vi "Dashboard Main.vi"() -> ()   [LabVIEW 2017]
uses:
  <vilib>/Utility/miscctls.llb/LVRowAndColumnTypeDef.ctl
  <vilib>/event_ctls.llb/eventvkey.ctl
  <vilib>/Rock Robotics/Network Tables/NT Read Numeric Array.vi
  <vilib>/Rock Robotics/WPI/Dashboard/WPI_DashboardLogging Global.vi
panel:
  in  "Camera Settings Right":T1={"Frame Rate"=30, "Compression"=30, "Size"=1, "DB Camera Config"=FALSE} {"Frame Rate" scale=1.0..30.0; "Compression" scale=100.0..-1.0; "Size" items=["640x480", "320x240", "160x120"]}
  in  "Camera Name Right":string(combo)="No Camera Selection"
  out "Camera Info":cluster{"Mbps LED":bool, "Mbps":dbl, "fps":dbl} {"fps" format="%#.1g"; "Mbps" format="%#.1g"}
  in  "Camera Settings":T1={"Frame Rate"=30, "Compression"=30, "Size"=1, "DB Camera Config"=FALSE} {"Frame Rate" scale=1.0..30.0; "Compression" scale=100.0..-1.0; "Size" items=["640x480", "320x240", "160x120"]}
  in  "TCP":refnum<k5>
  in  "Rec Mode":enum32{"Stop", "Record", "Playback"}(radio)
  out "Robot IP":string
  out "Image Message":string="Timeout in Camera Communications"
  in  "Dashboard Tab":T2(tab)
  in  "Select Auto":string(combo)="Select Autonomous ..."
  out "NT Connection":bool
  out "MotorChart R":cluster{"Numeric":dbl, "Numeric":dbl}(graph)
  out "MotorChart L":cluster{"Numeric":dbl, "Numeric":dbl}(graph)
  out "MotorSliders R":cluster{"MotorSlide1":dbl, "MotorSlide2":dbl} {"MotorSlide2" scale=-1.0..1.0 scale format="%#_2e"; "MotorSlide1" scale=-1.0..1.0 scale format="%#_2e"}
  out "MotorSliders L":cluster{"MotorSlide1":dbl, "MotorSlide2":dbl} {"MotorSlide2" scale=-1.0..1.0 scale format="%#_2e"; "MotorSlide1" scale=-1.0..1.0 scale format="%#_2e"}
  out "Gyro":dbl(knob) scale=0.0..360.0
  out "JS1 Z":dbl(slide) scale=-1.0..1.0 scale format="%#_2e"
  out "JS1 Graph":cluster{"X":dbl, "Y":dbl}[](graph)
  out "JS1 Buttons":T3
  out "JS2 Z":dbl(slide) scale=-1.0..1.0 scale format="%#_2e"
  out "JS2 Graph":cluster{"X":dbl, "Y":dbl}[](graph)
  out "JS2 Buttons":T3
  out "Mode":T4(ring)=enum."Auto Disabled"
  out "Game Specific Data":string
  out "Camera Image Right":T5(plugin-control)
  in  "DB/String 9":string
  in  "DB/String 8":string
  in  "DB/String 7":string
  in  "DB/String 6":string
  in  "DB/String 5":string
  in  "DB/String 4":string
  in  "DB/String 3":string
  in  "DB/String 2":string
  in  "DB/String 1":string
  in  "DB/String 0":string
  in  "DB/Slider 0":dbl(slide) scale=0.0..5.0
  in  "DB/Slider 1":dbl(slide) scale=0.0..5.0
  in  "DB/Slider 2":dbl(slide) scale=0.0..5.0
  in  "DB/Slider 3":dbl(slide) scale=0.0..5.0
  out "DB/LED 3":bool
  out "DB/LED 2":bool
  out "DB/LED 1":bool
  out "DB/LED 0":bool
  in  "DB/Button 3":bool
  in  "DB/Button 2":bool
  in  "DB/Button 1":bool
  in  "DB/Button 0":bool caption="New Name"
  in  "Test Tune":bool
  out "Array":bool[][](array[boolean])
  in  "Test Slider":dbl(slide) scale=0.0..100.0 scale format="%#_3g"
  in  "On/Off":bool caption="Solenoid"
  in  "Test Name":u16(ring) items=["Select the test to run..."]
  in  "Test Tree":string(tree)
  in  "Motor":cluster{"Value":dbl, "Enable":bool} {"Value" scale=-1.0..1.0 scale format="%#_3g"}
  out "Progress":T6 {"Test Progress" scale=0.0..100.0}
  in  "Rev/Fwd":cluster{"Forward":bool, "Reverse":bool}
  in  "Test Ring":u16(ring) items=["Monochrome", "Color"]
  out "Cmd Status":string
  in  "Execute Command":bool
  in  "Command Params":string[][](table)
  in  "Command Selection":i32(listbox)
  in  "CheckList":i32(listbox)
  out "Tree":string(tree)
  out "Camera Image":T5(plugin-control)
  out "Background":bool
  in  "Camera Name":string(combo)="No Camera Selection"
  # "HW"
  # "HW"
  # "Joysticks"
  # "Drive Motors"
  # "Front"
  # "Right"
  # "Left"
  # "Back"
  # "This tab is a great place for autonomous settings and robot-specific values.\nPlace controls and indicators inside this tab and match name to\nDashboard Variables on robot. You can also delete this comment."
  # "Opponent Switch\nScale\nOwn Switch"
  # "Left\nRight"
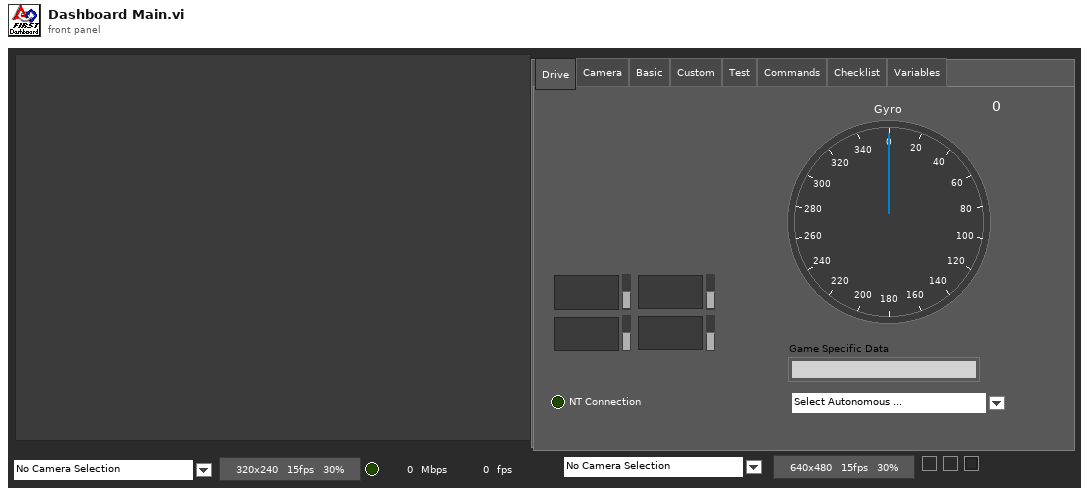
[diagram p1: front panel]
types:
  T1 = cluster{"Frame Rate":i32, "Compression":i32, "Size":u16, "DB Camera Config":bool}
  T2 = enum32{"Drive", "Camera", "Basic", "Custom", "Test", "Commands", "Checklist", "Variables"}
  T3 = cluster{bool, bool, bool, bool, bool, bool, bool, bool, bool, bool, bool, bool}
  T4 = enum8{"Tele-Op Disabled", "Tele-Op Enabled", "Auto Disabled", "Auto Enabled", "Test Disabled", "Test Enabled", "Disconnected", "No Code", "E-Stop"}
  T5 = typedef "IMAQ Image.ctl" = refnum<image>
  T6 = cluster{"Test Progress":u8, "Test Progress Text":string}
  T7 = cluster{"Save Path":path, "Interval (s)":dbl, "Keep":i32}
  T8 = typedef "Image Type" = u32
  T9 = cluster{"IDs":cluster{"RPC field ID":u16, "Unique ID":u16}, "String":string}
  T10 = cluster{"Error Strings":string, "Disable Counts":cluster{u16, u16}, "Rail Faults":cluster{u16, u16, u16}, "Robot IP":string, "DB Mode":u8, "Event Info":cluster{"Name":string, "Type":u8, "Number":u16, "Replay":u8}}
  T11 = cluster{"Storage":cluster{"Disk Free":u64, "RAM Block":u32, "RAM free":u32}, "CPU Utilization":cluster{"CPU % ISR":sgl, "CPU % Time Crit":sgl, "CPU % Timed Str":sgl, "CPU % High":sgl, "CPU % Above":sgl, "CPU % Normal":sgl, "CPU % Low":sgl}, "CAN":cluster{"% Bus Utilization":sgl, "Bus Off Cnt":u32, "TX_FIFO Full Cnt":u32, "Receive Error Cnt":u8, "Transmit Error Cnt":u8}, "HID":cluster{"HID Outputs":u32, "Rumble Low":u16, "Rumble High":u16}[]}
  T12 = cluster{"Status bits":cluster{"Test Mode":bool, "Autonomous":bool, "Enabled":bool, "Code Start":bool, "Brownout":bool, "Reserved 2":bool, "Reserved 3":bool, "E-Stop":bool}, "Code Trace":cluster{"Disabled":bool, "TeleOp":bool, "Auto":bool, "Test":bool}, "Controller Type":enum16{"unknown", "cRIO", "roboRio"}, "Code?":enum16{"unknown", "noCode", "code"}, "Battery V":dbl}
  T13 = cluster{"Control Bits":cluster{"TestMode":bool, "Autonomous":bool, "Enabled":bool, "FMS Present":bool, bool, bool, bool, "E-Stop":bool}, "Team Station ":u8, "Countdown":sgl, "Joystick Values":cluster{"Axes":dbl[], "Buttons":bool[], "POVs":i16[]}[]}
  T14 = cluster{"Axes":dbl[], "Buttons":bool[], "POVs":i16[]}[]
  T15 = cluster{"Axes":dbl[], "Buttons":bool[], "POVs":i16[]}
  T16 = cluster{"Buttons[0]":bool, "Buttons[1]":bool, "Buttons[2]":bool, "Buttons[3]":bool, "Buttons[4]":bool, "Buttons[5]":bool, "Buttons[6]":bool, "Buttons[7]":bool, "Buttons[8]":bool, "Buttons[9]":bool, "Buttons[10]":bool, "Buttons[11]":bool}
  T17 = cluster{"Camera Image":refnum<vi>, "Dashboard Tab":refnum<vi>, "Background":refnum<vi>, "Rec Mode":refnum<vi>, "Test Slider":refnum<vi>, "On/Off ":refnum<vi>, "Test Ring":refnum<vi>, "Rev/Fwd":refnum<vi>, "Test Name":refnum<vi>, "Motor":refnum<vi>, "Progress":refnum<vi>, "CheckList":refnum<vi>, "Tree":refnum<vi>, "Test Tree":refnum<vi>, "Command Params":refnum<vi>, "Command Selection":refnum<vi>, "Execute Command":refnum<vi>, "Cmd Status":refnum<vi>, "Camera Settings":refnum<vi>, "Camera Name":refnum<vi>, "Camera Info":refnum<vi>, "Camera Settings Right":refnum<vi>, "Camera Name Right":refnum<vi>, "Camera Image Right":refnum<vi>}
  T18 = cluster{"Camera Name":string, string, "Saved DB Images Info":cluster{"Save Path":path, "Interval (s)":dbl, "Keep":i32}}
  T19 = cluster{"Camera Name Right":string, string, "Saved DB Images Info":cluster{"Save Path":path, "Interval (s)":dbl, "Keep":i32}}
  T20 = cluster{"Operation":enum16{"Update", "Clear"}, "Color Box":u32}[]
  T21 = typedef "eventvkey.ctl" = enum16{"ASCII", "Enter", "Return", "Shift", "Ctrl", "Alt", "Cmd", "Opt", "Caps", "NumLock", "Clear", "Break", "Up", "Down", "Left", "Right", "Insert", "Delete", "Home", "End", "PageUp", "PageDown", "Escape", "Help", "Pause", "ScrollLock", "F1", "F2", "F3", "F4", "F5", "F6", "F7", "F8", "F9", "F10", "F11", "F12", "F13", "F14", "F15", "F16", "F17", "F18", "F19", "F20", "F21", "F22", "F23", "F24", "Play", "VolumeUp", "VolumeDown", "Mute", "Two Byte Char"}
  T22 = cluster{"Image Size":bool, "Image Type":bool, "Pixel Value":bool, "ROI Information":bool, "Zoom Factor":bool}
  T23 = cluster{"Operation":enum16{"Update", "Clear"}, "Color Box":u32}
  T24 = typedef "LVRowAndColumnTypeDef.ctl" = cluster{"Row":i32, "Column":i32}
  T25 = cluster{"Shift":bool, "Ctrl":bool, "Alt":bool, "Cmd":bool, "Opt":bool}
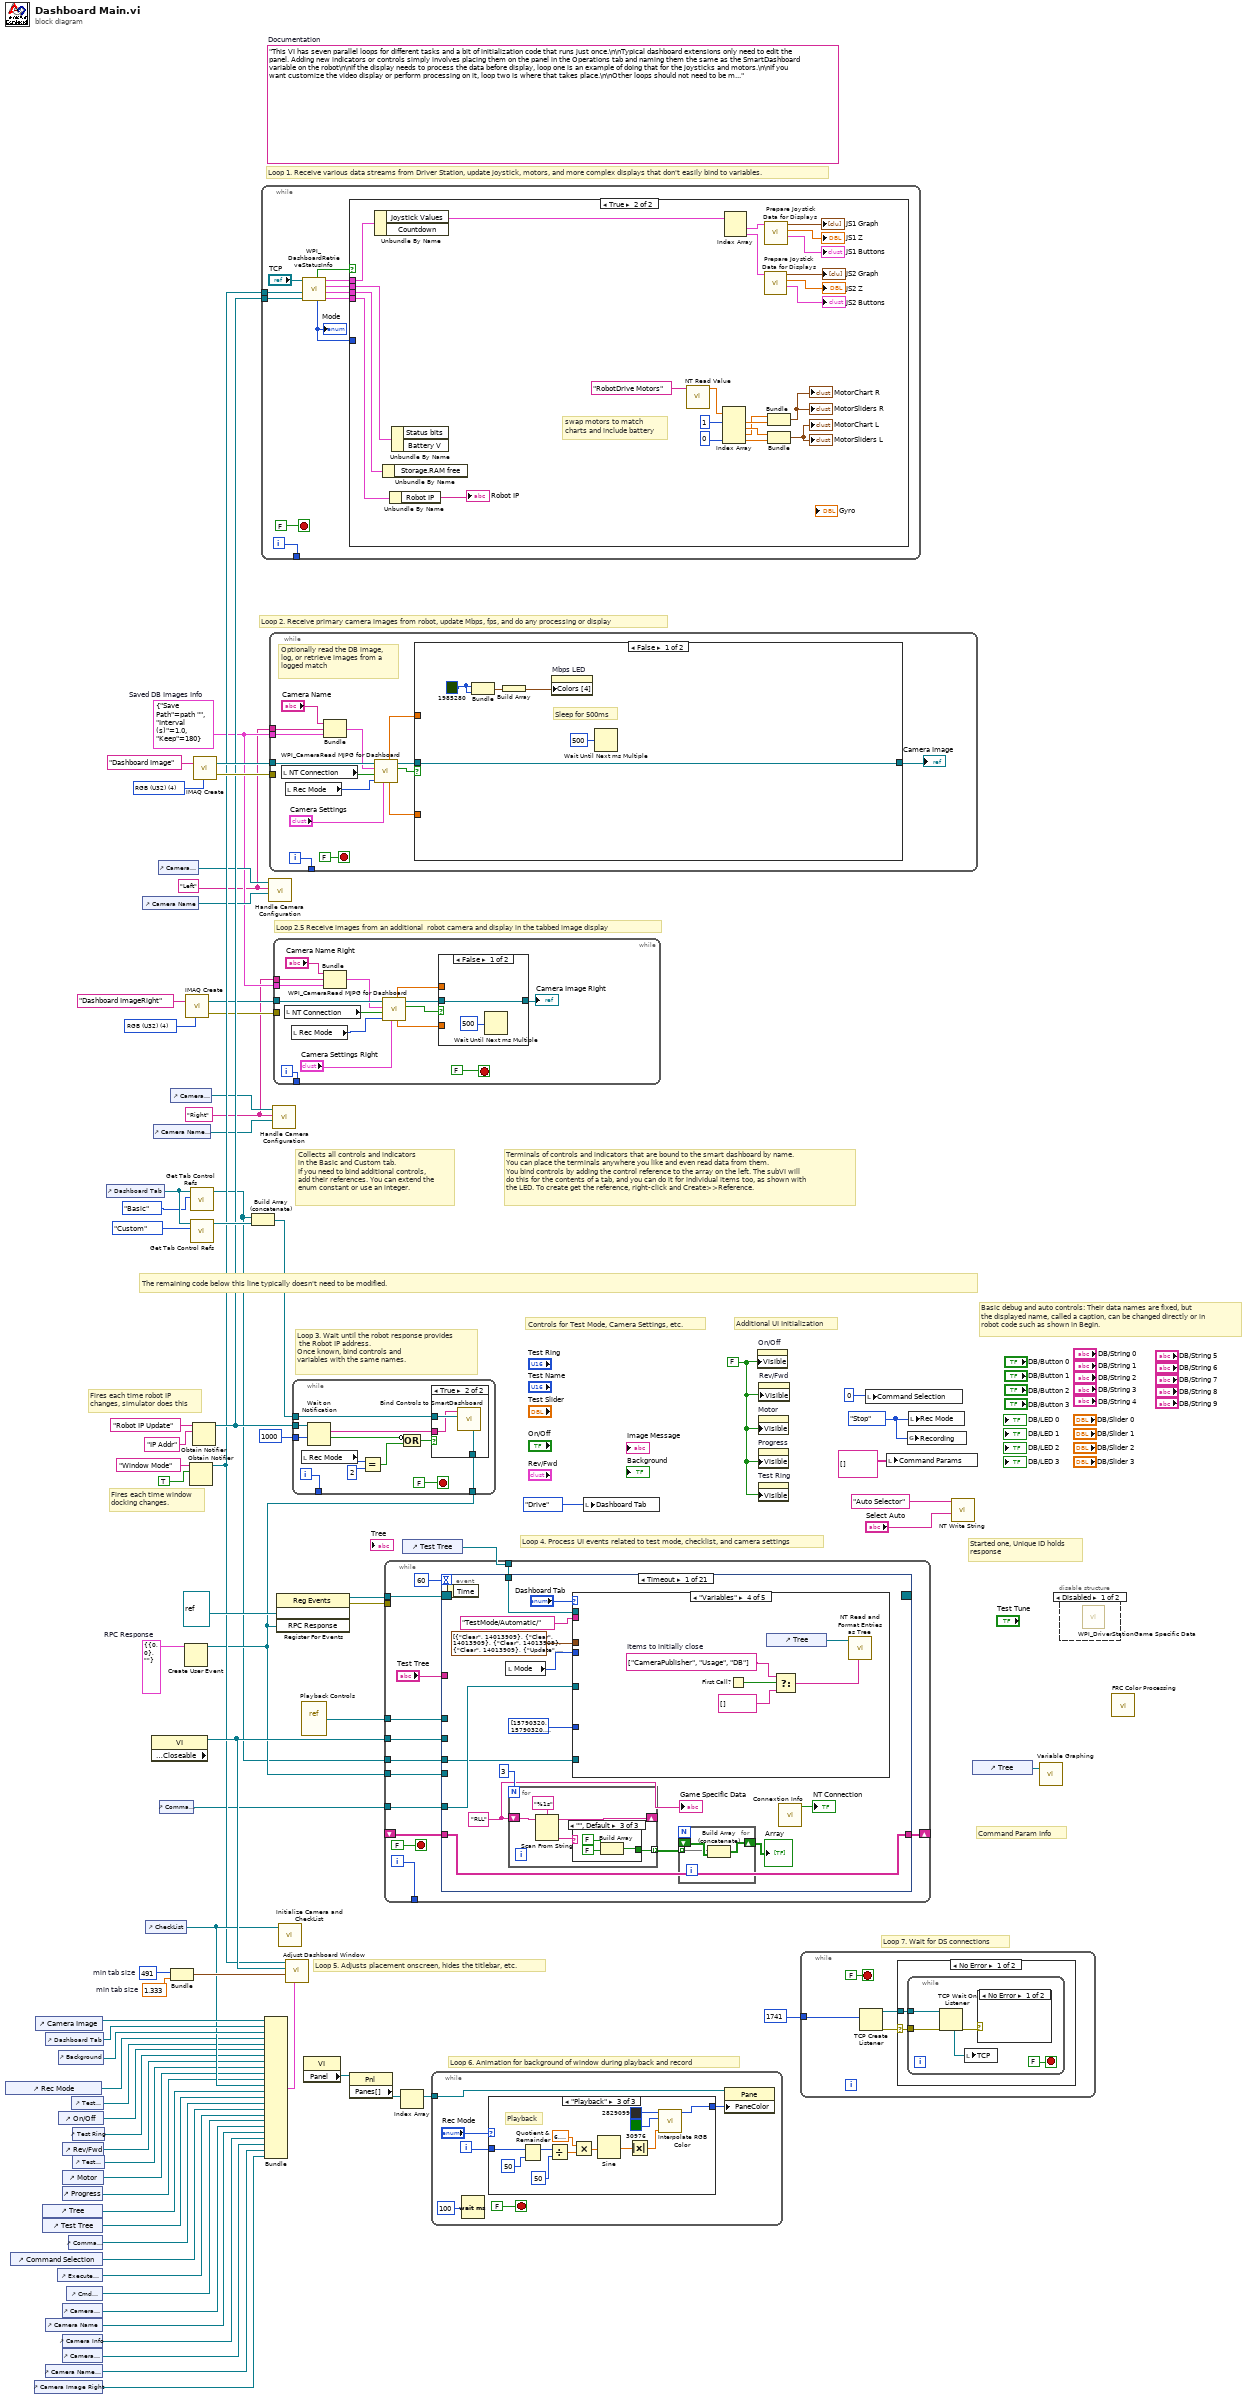
[diagram p0: block diagram]
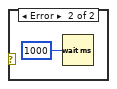
[diagram p4: hidden frame]
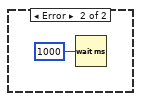
[diagram p5: hidden frame]
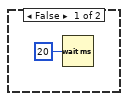
[diagram p6: hidden frame]
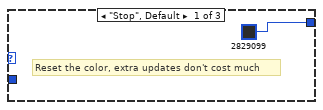
[diagram p7: hidden frame]
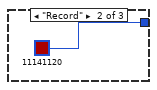
[diagram p8: hidden frame]
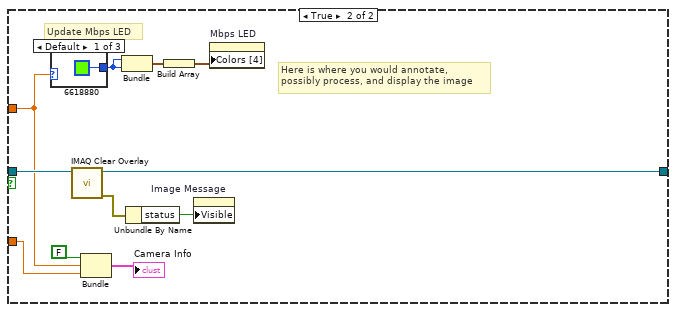
[diagram p10: hidden frame]
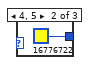
[diagram p11: hidden frame]
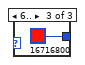
[diagram p12: hidden frame]
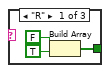
[diagram p13: hidden frame]
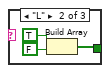
[diagram p14: hidden frame]
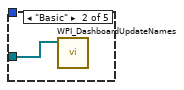
[diagram p16: hidden frame]
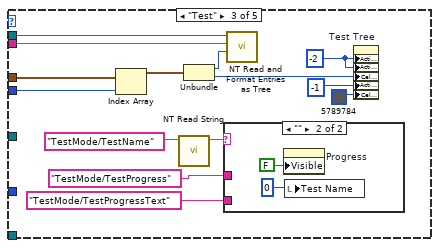
[diagram p17: hidden frame]
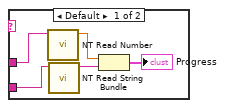
[diagram p18: hidden frame]
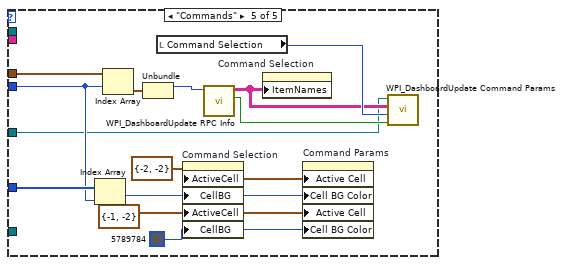
[diagram p19: hidden frame]
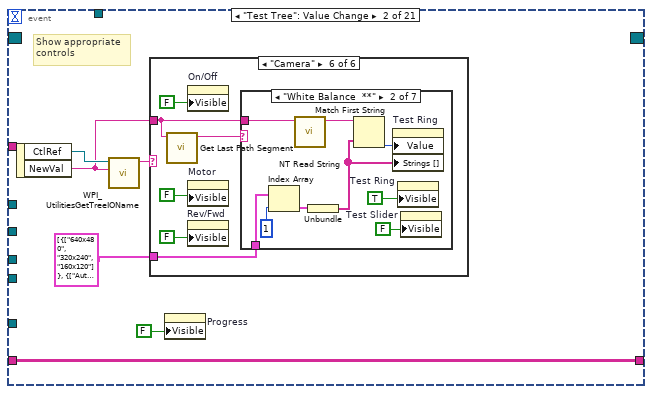
[diagram p20: hidden frame]
diagram:
  w4 = T7 {"Save Path"=path "", "Interval (s)"=1.0, "Keep"=180}  # Saved DB Images Info
  w3 = "Right"
  w2 = "Left"
  w14 = T8 4 items=["Grayscale (U8)", "Grayscale (I16)", "Grayscale (SGL)", "Complex (CSG)", "RGB (U32)", "HSL (U32)", "RGB (U64)"] ("Image Type")
  w30 = T9 {"IDs"={"RPC field ID"=0, "Unique ID"=0}, "String"=""}  # RPC Response
  w53 = 491  # min tab size
  w52 = 1.333  # min tab size
  w60 = enum32{"Stop", "Record", "Playback"}."Stop" ("Rec Mode")
  w37 = FALSE ("Visible")
  (unwired) "This VI has seven parallel loops for different tasks and a bit of initialization code that runs just once.\n\nTypical dashboard extensions only need to edit the panel. Adding new indicators or controls simply involves placing them on the panel in the Operations tab and naming them the same as the SmartDashboard variable on the robot\n\nIf the display needs to process the data before display, loop one is an example of doing that for the joysticks and motors.\n\nIf you want customize the video display or perform processing on it, loop two is where that takes place.\n\nOther loops should not need to be modified. They are pretty standard, and document the task they perform."  # Documentation
  w77 = T8 4 items=["Grayscale (U8)", "Grayscale (I16)", "Grayscale (SGL)", "Complex (CSG)", "RGB (U32)", "HSL (U32)", "RGB (U64)"] ("Image Type")
  # "Loop 2.5 Receive images from an additional  robot camera and display in the tabbed image display"
  # "Command Param Info"
  # "Started one, Unique ID holds\nresponse"
  # "Loop 7. Wait for DS connections"
  # "Basic debug and auto controls: Their data names are fixed, but\nthe displayed name, called a caption, can be changed directly or in\nrobot code such as shown in Begin."
  # "Controls for Test Mode, Camera Settings, etc."
  # "Additional UI Initialization"
  # "Loop 6. Animation for background of window during playback and record"
  # "Fires each time robot IP\nchanges, simulator does this"
  # "Fires each time window\ndocking changes."
  # "Collects all controls and indicators\nin the Basic and Custom tab.\nIf you need to bind additional controls,\nadd their references. You can extend the\nenum constant or use an integer."
  # "The remaining code below this line typically doesn't need to be modified."
  # "Loop 4. Process UI events related to test mode, checklist, and camera settings"
  # "Terminals of controls and indicators that are bound to the smart dashboard by name.\nYou can place the terminals anywhere you like and even read data from them.\nYou bind controls by adding the control reference to the array on the left. The subVI will\ndo this for the contents of a tab, and you can do it for individual items too, as shown with\nthe LED. To create get the reference, right-click and Create>>Reference."
  # "Loop 3. Wait until the robot response provides\n the Robot IP address.\nOnce known, bind controls and\nvariables with the same names."
  # "Loop 5. Adjusts placement onscreen, hides the titlebar, etc."
  # "Loop 1. Receive various data streams from Driver Station, update joystick, motors, and more complex displays that don't easily bind to variables."
  # "Loop 2. Receive primary camera images from robot, update Mbps, fps, and do any processing or display"
  n1 = control-ref of="Rec Mode"() -> (w43:refnum<vi>)
  n2 = control-ref of="Command Selection"() -> (w29:refnum<vi>)
  n3 = control-ref of="Camera Image Right"() -> (w7:refnum<vi>)
  n4 = control-ref of="Camera Image"() -> (w55:refnum<vi>)
  n5 = control-ref of="Tree"() -> (w47:refnum<vi>)
  n6 = control-ref of="Test Tree"() -> (w46:refnum<vi>)
  n7 = control-ref of="Dashboard Tab"() -> (w54:refnum<vi>)
  n8 = control-ref of="Camera Name"() -> (w20:refnum<vi>)
  n9 = control-ref of="Camera Name Right"() -> (w8:refnum<vi>)
  n10 = control-ref of="Execute Command"() -> (w31:refnum<vi>)
  n11 = control-ref of="Background"() -> (w50:refnum<vi>)
  n12 = control-ref of="On/Off"() -> (w41:refnum<vi>)
  n13 = control-ref of="Progress"() -> (w38:refnum<vi>)
  n14 = control-ref of="Camera Settings"() -> (w21:refnum<vi>)
  n15 = control-ref of="Camera Info"() -> (w19:refnum<vi>)
  n16 = control-ref of="Camera Settings Right"() -> (w9:refnum<vi>)
  n17 = control-ref of="Rev/Fwd"() -> (w39:refnum<vi>)
  n18 = control-ref of="Motor"() -> (w44:refnum<vi>)
  n19 = control-ref of="Cmd Status"() -> (w25:refnum<vi>)
  n20 = control-ref of="Command Params"() -> (w32:refnum<vi>)
  n21 = control-ref of="Test Slider"() -> (w42:refnum<vi>)
  n22 = control-ref of="Test Ring"() -> (w40:refnum<vi>)
  n23 = control-ref of="Test Name"() -> (w45:refnum<vi>)
  n24 = control-ref of="Dashboard Tab"() -> (w58:refnum<vi>)
  n25 = control-ref of="Camera Name"() -> (w22:refnum<vi>)
  n26 = control-ref of="CheckList"() -> (w48:refnum<vi>)
  n27 = property class="VI" props=["Front Panel.Closeable"]() -> (reference out=w59:refnum<vi>)  [unwired: 2 in, 2 out]
  n28 = control-ref of="Camera Name Right"() -> (w10:refnum<vi>)
  n29 = control-ref of="Camera Settings"() -> (w23:refnum<vi>)
  n30 = control-ref of="Command Params"() -> (w24:refnum<vi>)
  n31 = control-ref of="Camera Settings Right"() -> (w11:refnum<vi>)
  n32 = Bundle("min tab size"=w53, "min tab size"=w52) -> (w51:cluster{"min tab size":i32, "min tab size":dbl})  [unwired: 1 in]
  n33 = Create User Event(user event datatype=w30) -> (user event=w26:refnum<user-event>)  [unwired: 1 in, 1 out]
  n34 = call "IMAQ Create"("Image Name"="Dashboard ImageRight", "Image Type"=w14) -> ("New Image"=w13:T5, "error out"=w12:errorcluster)  [unwired: 2 in, 1 out]
  n35 = Obtain Notifier(name (unnamed)="Window Mode", notification data type=TRUE) -> (notifier out=w35:refnum<notifier>)  [unwired: 2 in, 2 out]
  n36 = call <vilib>:"Get Tab Control Refs.vi"("Page Index"=T2."Basic" ("Dashboard Tab"), "TabControl in"=w58) -> ("ControlsOnPage"=w18:refnum<vi>[])  [unwired: 9 in]
  n37 = call <vilib>:"Get Tab Control Refs.vi"("Page Index"=T2."Custom" ("Dashboard Tab"), "TabControl in"=w58) -> ("ControlsOnPage"=w57:refnum<vi>[])  [unwired: 9 in]
  n38 = Obtain Notifier(name (unnamed)="Robot IP Update", notification data type="IP Addr" ("name (unnamed)")) -> (notifier out=w36:refnum<notifier>)  [unwired: 2 in, 2 out]
  n39 = call "IMAQ Create"("Image Name"="Dashboard Image", "Image Type"=w77) -> ("New Image"=w75:T5, "error out"=w74:errorcluster)  [unwired: 2 in, 1 out]
  n40 = Build Array (concatenate)(w18, w57) -> (w56:refnum<vi>[])
  n41 = while {
    tunnel: [w87] -> _
    tunnel: w36 -> [w81]
    tunnel: w35 -> [w78]
    i -> [w87]
    stop <- FALSE stop-if-true
    n42 = call <vilib>:"WPI_DashboardRetrieveStatusInfo.vi"("Binding Refnum"=w81, "Window Mode Notifier"=w78, "TCP Cnx"="TCP") -> ("Power and Errors"=w82:T10, "Robot Metrics"=w85:T11, "Status Info"=w86:T12, "Control Info"=w83:T13, "Robot Mode"=w80:T4, "Process?"=w84:bool)  [unwired: 3 in]
    "Mode" <- w80
    n43 = case shown="True" w84 {
      tunnel: w86 -> [_ w113]
      tunnel: w85 -> [_ w112]
      tunnel: w83 -> [_ w111]
      tunnel: w82 -> [_ w110]
      tunnel: w80 -> [_ _]
      frame False {
        n44 = Wait (ms)(milliseconds to wait=u32 20) -> ()  [unwired: 1 out]
      }
      frame True {
        # "swap motors to match\ncharts and include battery"
        n45 = Unbundle By Name(w111) -> ("Joystick Values"=w101:T14)  [unwired: 1 out]
        n46 = Unbundle By Name(w112) -> ()  [unwired: 1 out]
        n47 = Unbundle By Name(w110) -> ("Robot IP"=→"Robot IP":string)
        n48 = Unbundle By Name(w113) -> ()  [unwired: 2 out]
        n49 = call-poly <vilib>:"NT Read Value.vi"("Name"="RobotDrive Motors") -> ("Numeric Array"=w91:dbl[])  [unwired: 9 in, 1 out]
        n50 = Index Array(array=w91, index #1=1, index #4=0) -> (element #1=w105:dbl, element #2=w106:dbl, element #3=w104:dbl, element #4=w109:dbl)  [unwired: 2 in]
        n51 = Index Array(array=w101) -> (element #1=w100:T15, element #2=w96:T15)  [unwired: 2 in]
        n52 = call "Prepare Joystick Data for Displays.vi"("Joystick Values"=w96) -> ("Buttons"=→"JS2 Buttons":T16, "Z Axis"=→"JS2 Z":dbl, "Cartesian Data"=→"JS2 Graph":cluster{"X axis":dbl, "X axis":dbl}[])  [unwired: 8 in]
        n53 = call "Prepare Joystick Data for Displays.vi"("Joystick Values"=w100) -> ("Buttons"=→"JS1 Buttons":T16, "Z Axis"=→"JS1 Z":dbl, "Cartesian Data"=→"JS1 Graph":cluster{"X axis":dbl, "X axis":dbl}[])  [unwired: 8 in]
        n54 = Bundle("Numeric"=w104, "Numeric"=w105) -> (→"MotorChart R" →"MotorSliders R":cluster{"Numeric":dbl, "Numeric":dbl})  [unwired: 1 in]
        n55 = Bundle("Numeric"=w106, "Numeric"=w109) -> (→"MotorChart L" →"MotorSliders L":cluster{"Numeric":dbl, "Numeric":dbl})  [unwired: 1 in]
      }
    }
  }
  n56 = Bundle("Camera Image"=w55, "Dashboard Tab"=w54, "Background"=w50, "Rec Mode"=w43, "Test Slider"=w42, "On/Off"=w41, "Test Ring"=w40, "Rev/Fwd"=w39, "Test Name"=w45, "Motor"=w44, "Progress"=w38, "CheckList"=w48, "Tree"=w47, "Test Tree"=w46, "Command Params"=w32, "Command Selection"=w29, "Execute Command"=w31, "Cmd Status"=w25, "Camera Settings"=w21, "Camera Name"=w20, "Camera Info"=w19, "Camera Settings Right"=w9, "Camera Name Right"=w8, "Camera Image Right"=w7) -> (w49:T17)  [unwired: 1 in]
  n57 = call "Handle Camera Configuration.vi"("CameraNameRef"=w22, "Display Name"=w2, "ClusterRef"=w23) -> ()  [unwired: 9 in]
  n58 = while {
    tunnel: w75 -> [w126]
    tunnel: w74 -> [_]
    tunnel: [w127] -> _
    tunnel: w4 -> [w117]
    tunnel: w2 -> [w114]
    i -> [w127]
    stop <- FALSE stop-if-true
    # "Optionally read the DB image,\nlog, or retrieve images from a\nlogged match"
    n59 = local read "NT Connection"() -> (w118:bool)
    n60 = local read "Rec Mode"() -> (w122:enum32{"Stop", "Record", "Playback"})
    n61 = Bundle("Camera Name"="Camera Name", w114, "Saved DB Images Info"=w117) -> (w116:T18)  [unwired: 1 in]
    n62 = call <vilib>:"WPI_CameraRead MJPG for Dashboard.vi"("Camera Settings"="Camera Settings", "Rec Mode"=w122, "NT Connection"=w118, "Capture Info"=w116, "Refnum in"=w126) -> ("Active"=w124:bool, "Refnum out"=w125:T5, "FPS"=w123:dbl, "Bandwidth (Mbps)"=w121:dbl)  [unwired: 3 in]
    n63 = case shown="False" w124 {
      tunnel: w125 -> [w129 w140]
      tunnel: w121 -> [_ w137]
      tunnel: w123 -> [_ w138]
      tunnel: [w129 w134] -> w119
      frame False {
        w131 = u32 1985280 ("Color Box")
        # "Sleep for 500ms"
        n64 = Bundle("Color Box"=w131, "Color Box"=w131) -> (w132:cluster{"Color Box":u32, "Color Box":u32})  [unwired: 1 out]
        n65 = Build Array(w132) -> (w130:cluster{"Color Box":u32, "Color Box":u32}[])
        n66 = property on="Mbps LED" class="Bool (strict)"("Colors [4]"=w130) -> ()  [unwired: 2 in, 2 out]
        n67 = Wait Until Next ms Multiple(millisecond multiple=u32 500) -> ()  [unwired: 1 out]
      }
      frame True {
        # "Here is where you would annotate,\npossibly process, and display the image"
        # "Update Mbps LED"
        n68 = case shown="Default" w137 {
          tunnel: [u32 6618880 ("Color Box") u32 16776722 ("Color Box") u32 16716800 ("Color Box")] -> w141
          frame Default {
          }
          frame 4, 5 {
          }
          frame 6.. {
          }
        }
        n69 = call "IMAQ Clear Overlay"("Image"=w140) -> ("error out"=w143:errorcluster, "Image Out"=w134:T5)  [unwired: 2 in, 7 out]
        n70 = Bundle(FALSE, "Bandwidth (Mbps)"=w137, "FPS"=w138) -> (→"Camera Info":cluster{bool, "Bandwidth (Mbps)":dbl, "FPS":dbl})  [unwired: 1 in]
        n71 = Bundle("Color Box"=w141, "Color Box"=w141) -> (w142:cluster{"Color Box":u32, "Color Box":u32})  [unwired: 1 out]
        n72 = Unbundle By Name(w143) -> ("status"=w144:bool)
        n73 = Build Array(w142) -> (w139:cluster{"Color Box":u32, "Color Box":u32}[])
        n74 = property on="Image Message" class="Str"("Visible"=w144) -> ()  [unwired: 2 in, 2 out]
        n75 = property on="Mbps LED" class="Bool (strict)"("Colors [4]"=w139) -> ()  [unwired: 2 in, 2 out]
      }
    }
    "Camera Image" <- w119
  }
  n76 = call "Handle Camera Configuration.vi"("CameraNameRef"=w10, "Display Name"=w3, "ClusterRef"=w11) -> ()  [unwired: 9 in]
  n77 = while {
    tunnel: w13 -> [w162]
    tunnel: w12 -> [_]
    tunnel: [w157] -> _
    tunnel: w4 -> [w151]
    tunnel: w3 -> [w148]
    i -> [w157]
    stop <- FALSE stop-if-true
    n78 = local read "NT Connection"() -> (w152:bool)
    n79 = local read "Rec Mode"() -> (w161:enum32{"Stop", "Record", "Playback"})
    n80 = Bundle("Camera Name Right"="Camera Name Right", w148, "Saved DB Images Info"=w151) -> (w150:T19)  [unwired: 1 in]
    n81 = call <vilib>:"WPI_CameraRead MJPG for Dashboard.vi"("Camera Settings"="Camera Settings Right", "Rec Mode"=w161, "NT Connection"=w152, "Capture Info"=w150, "Refnum in"=w162) -> ("Active"=w156:bool, "Refnum out"=w159:T5, "FPS"=w154:dbl, "Bandwidth (Mbps)"=w155:dbl)  [unwired: 3 in]
    n82 = case shown="False" w156 {
      tunnel: w159 -> [w163 w165]
      tunnel: w155 -> [_ _]
      tunnel: w154 -> [_ _]
      tunnel: [w163 w165] -> w153
      frame False {
        n83 = Wait Until Next ms Multiple(millisecond multiple=u32 500) -> ()  [unwired: 1 out]
      }
      frame True {
      }
    }
    "Camera Image Right" <- w153
  }
  n84 = register-events(refnum<vi> refnum, w26) -> (reference out=w64:refnum<event-registration>, error out=w63:errorcluster)  [unwired: 2 in]
  n85 = call "Initialize Camera and CheckList.vi"("ListBox in"=w48) -> ()  [unwired: 11 in]
  n86 = call "Adjust Dashboard Window.vi"("Sizing Refnums"=w49, "Size Constraints"=w51, "VI"=w59, "WIn Mode"=w35) -> ()  [unwired: 8 in]
  n87 = while {
    tunnel: w56 -> [w177]
    tunnel: w36 -> [w175]
    tunnel: [w173] -> _
    tunnel: u32 1000 ("milliseconds to wait") -> [w172]
    tunnel: w26 -> [w166]
    i -> [w173]
    stop <- FALSE stop-if-true
    n88 = local read "Rec Mode"() -> (w168:enum32{"Stop", "Record", "Playback"})
    n89 = Wait on Notification(notifier=w175, timeout in ms (-1)=w172) -> (notification=w174:string, timed out?=w170:bool)  [unwired: 2 in, 2 out]
    n90 = Equal?(x=w168, y=u16 2 ("Rec Mode")) -> (x = y?=w169:bool)
    n91 = Compound Arithmetic op=OR(invert w170, w169) -> (w171:bool)
    n92 = case shown="True" w171 {
      tunnel: w177 -> [_ w180]
      tunnel: w174 -> [_ w179]
      tunnel: w166 -> [_ w178]
      frame False {
      }
      frame True {
        n93 = call <vilib>:"Bind Controls to SmartDashboard.vi"("RPC ref"=w178, "Bound Control Refs"=w180, "Server IP Address"=w179) -> ()  [unwired: 9 in]
      }
    }
  }
  n94 = vi-ref "Playback Controls.vi"() -> (w65:refnum<vi>)
  n95 = property class="VI"() -> ("Panel"=w67:refnum<vi>)  [unwired: 2 in, 2 out]
  n96 = property class="Pnl"(reference=w67) -> ("Panes[]"=w68:refnum<vi>[])  [unwired: 1 in, 2 out]
  n97 = Index Array(array=w68) -> (element=w66:refnum<vi>)  [unwired: 1 in]
  n98 = control-ref of="Test Tree"() -> (w69:refnum<vi>)
  n99 = while {
    tunnel: [w190] -> _
    tunnel: w69 -> [w189]
    tunnel: w65 -> [w188]
    tunnel: w64 -> [w187]
    tunnel: w63 -> [_]
    tunnel: w59 -> [w186]
    tunnel: w26 -> [w185]
    tunnel: w24 -> [w184]
    shift-right: [w183] -> _
    shift-left: _ -> [w182]
    tunnel: w18 -> [w181]
    i -> [w190]
    stop <- FALSE stop-if-true
    n100 = event shown="[0] Timeout" {
      selector: w187 -> [_ _ _ _ _ _ _ _ _ _ _ _ _ _ _ _ _ _ _ _ _]
      dyn-events: [_ _ _ _ _ _ _ _ _ _ _ _ _ _ _ _ w471 _ _ _ _] -> _
      timeout: u32 60 ("milliseconds to wait") -> [_ _ _ _ _ _ _ _ _ _ _ _ _ _ _ _ _ _ _ _ _]
      tunnel: w189 -> [w206 _ _ _ _ _ _ _ _ _ _ _ _ _ _ _ _ _ _ _ _]
      tunnel: "Test Tree" -> [_ _ _ _ _ _ _ _ _ _ _ w438 w446 w448 w452 w460 _ _ _ _ _]
      tunnel: w188 -> [_ _ _ _ _ _ _ _ _ _ _ _ _ _ _ _ w473 _ w491 _ _]
      tunnel: w186 -> [_ _ _ _ _ _ _ _ _ _ _ _ _ _ _ _ w469 _ _ _ _]
      tunnel: w185 -> [_ _ _ _ _ _ _ _ _ _ _ _ _ _ _ _ w467 _ _ _ _]
      tunnel: w184 -> [w201 _ _ _ _ _ w389 _ _ _ _ _ _ _ _ _ _ _ _ _ _]
      tunnel: [w200 w266 w368 w373 w382 w386 w387 w396 w406 w413 w425 w437 w444 w447 w451 w459 w466 w486 w488 w492 w505] -> w183
      tunnel: w182 -> [w200 w266 w368 w373 w382 w386 w387 _ _ w413 w425 w437 w444 w447 w451 w459 w466 w486 w488 w492 w505]
      tunnel: w181 -> [w198 _ _ _ _ _ _ _ _ _ _ _ _ _ _ _ _ _ _ _ _]
      event Timeout {
        w196 = "RLL" ("Game Specific Data")
        n101 = event-data() -> ()  [unwired: 1 in, 1 out]
        n102 = local read "Mode"() -> (w203:T4)
        n103 = for {
          N: 3 -> [_]
          shift-right: [w211] -> _
          shift-left: w196 -> [w215]
          tunnel: [w212] -> w195 mode=indexing
          n104 = Scan From String(format string="%1s", input string=w215) -> (remaining string=w211:string, output 1=w213:string)  [unwired: 3 in, 2 out]
          n105 = case shown="\"\", Default" w213 {
            tunnel: [w216 w219 w222] -> w212
            frame "R" {
              n106 = Build Array(FALSE, TRUE) -> (w216:bool[])
            }
            frame "L" {
              n107 = Build Array(TRUE, FALSE) -> (w219:bool[])
            }
            frame "", Default {
              n108 = Build Array(FALSE, FALSE) -> (w222:bool[])
            }
          }
        }
        n109 = case shown="\"Variables\"" "Dashboard Tab" {
          tunnel: w206 -> [_ _ w239 _ _]
          tunnel: "TestMode/Automatic/" ("Name Pattern") -> [_ _ w238 _ _]
          tunnel: T20 [{"Operation"=enum."Clear", "Color Box"=14013909}, {"Operation"=enum."Clear", "Color Box"=14013909}, {"Operation"=enum."Clear", "Color Box"=14013909}, {"Operation"=enum."Clear", "Color Box"=14013909}, {"Operation"=enum."Update", "Color Box"=14013909}, {"Operation"=enum."Update", "Color Box"=16777215}, {"Operation"=enum."Clear", "Color Box"=14013909}, {"Operation"=enum."Clear", "Color Box"=14013909}, {"Operation"=enum."Clear", "Color Box"=14013909}] -> [_ _ w231 _ w259]
          tunnel: w203 -> [_ _ w230 _ w258]
          tunnel: u32[] [15790320, 15790320, 15790320, 15790320, 16777215, 16777215, 15790320, 15790320, 15790320] -> [_ _ _ _ w264]
          tunnel: w201 -> [_ _ _ _ w252]
          tunnel: w198 -> [_ w225 _ _ _]
          frame "Custom", Default {
          }
          frame "Basic" {
            n110 = call <vilib>:"WPI_DashboardUpdateNames.vi"("Controls on Tab"=w225) -> ()  [unwired: 11 in]
          }
          frame "Test" {
            w237 = -2 ("Active Item:Row Number")
            n111 = Index Array(array=w231, index=w230) -> (element=w232:T23)
            n112 = call <vilib>:"NT Read String.vi"("Name"="TestMode/TestName") -> ("String"=w228:string)  [unwired: 9 in, 1 out]
            n113 = Unbundle(w232) -> ("Operation"=w233:enum16{"Update", "Clear"}, "Color Box"=w234:u32)
            n114 = case shown="\"\"" w228 {
              tunnel: "TestMode/TestProgress" ("Name") -> [w241 _]
              tunnel: "TestMode/TestProgressText" ("Name") -> [w240 _]
              frame Default {
                n115 = call <vilib>:"NT Read Number.vi"("Name"=w241) -> ("Numeric"=w242:dbl)  [unwired: 9 in, 1 out]
                n116 = call <vilib>:"NT Read String.vi"("Name"=w240) -> ("String"=w243:string)  [unwired: 9 in, 1 out]
                n117 = Bundle("Numeric"=w242, "String"=w243) -> (→"Progress":cluster{"Numeric":dbl, "String":string})  [unwired: 1 in]
              }
              frame "" {
                n118 = property on="Progress" class="Clust (strict)"("Visible"=FALSE) -> ()  [unwired: 2 in, 2 out]
                n119 = local write "Test Name"(u16 0) -> ()
              }
            }
            n120 = call <vilib>:"NT Read and Format Entries as Tree.vi"("Operation"=w233, "Name Pattern"=w238, "Tree Refnum"=w239) -> ()  [unwired: 7 in, 2 out]
            n121 = property on="Test Tree" class="Tree (strict)"("Active Item Row Number"=w237, "ActiveColNum"=w237, "CellBG"=w234, "Active Item Row Number"=-1 ("Active Item:Row Number"), "CellBG"=u32 5789784 ("Color Box")) -> ()  [unwired: 2 in, 2 out]
          }
          frame "Variables" {
            w249 = string[] ["CameraPublisher", "Usage", "DB"]  # Items to initially close
            n122 = First Call?() -> (First Call?: T/F=w250:bool)
            n123 = control-ref of="Tree"() -> (w251:refnum<vi>)
            n124 = Select(t=w249, s=w250, f=string[] []) -> (s? t:f=w247:string[])
            n125 = call <vilib>:"NT Read and Format Entries as Tree.vi"("Tags to  Close"=w247, "Tree Refnum"=w251) -> ()  [unwired: 8 in, 2 out]
          }
          frame "Commands" {
            w260 = u32 5789784 ("Color Box")
            w261 = T24 {"Row"=-1, "Column"=-2} ("Active Cell:Active Cell")
            w263 = T24 {"Row"=-2, "Column"=-2} ("Active Cell:Active Cell")
            n126 = Index Array(array=w264, index=w258) -> (element=w262:u32)
            n127 = Index Array(array=w259, index=w258) -> (element=w257:T23)
            n128 = Unbundle(w257) -> ("Operation"=w256:enum16{"Update", "Clear"})  [unwired: 1 out]
            n129 = local read "Command Selection"() -> (w255:i32)
            n130 = property on="Command Selection" class="MCListbox (strict)"("ActiveCell"=w263, "CellBG"=w262, "ActiveCell"=w261, "CellBG"=w260) -> ()  [unwired: 2 in, 2 out]
            n131 = call <vilib>:"WPI_DashboardUpdate RPC Info.vi"("Operation"=w256) -> ("update"=w254:bool, "commands"=w253:string[][])  [unwired: 9 in]
            n132 = property on="Command Selection" class="MCListbox (strict)"("ItemNames"=w253) -> ()  [unwired: 2 in, 2 out]
            n133 = property on="Command Params" class="Tbl (strict)"("Active Cell"=w263, "Cell BG Color"=w262, "Active Cell"=w261, "Cell BG Color"=w260) -> ()  [unwired: 2 in, 2 out]
            n134 = call <vilib>:"WPI_DashboardUpdate Command Params.vi"("Update"=w254, "NewVal"=w255, "Commands"=w253, "Param Tbl"=w252) -> ()  [unwired: 7 in, 1 out]
          }
        }
        n135 = for {
          tunnel: w195 -> [w208] mode=indexing
          shift-right: [w210] -> w194
          shift-left: _ -> [w209]
          n136 = Build Array (concatenate)(w208, w209) -> (w210:bool[][])
        }
        "Array" <- w194
        n137 = call <vilib>:"Connextion Info.vi"() -> ("Connected"=→"NT Connection":bool)  [unwired: 10 in, 1 out]
        "Game Specific Data" <- w196
      }
      event "Test Tree": Value Change {
        # "Show appropriate\ncontrols"
        n138 = event-data() -> ("CtlRef"=w269:refnum<vi>, "NewVal"=w267:string)  [unwired: 1 in]
        n139 = call <vilib>:"WPI_UtilitiesGetTreeIOName.vi"("NewVal"=w267, "TreeControl in"=w269) -> ("I/O Name"=w270:string)  [unwired: 9 in]
        n140 = case shown="\"Camera\"" w270 {
          selector: w270 -> [_ w277 _ w299 w308 _]
          tunnel: w267 -> [_ _ w296 w298 _ w315]
          tunnel: cluster{string[]}[] [{["640x480", "320x240", "160x120"]}, {["Auto", "Fixed indoor", "Fixed outdoor 1", "Fixed outdoor 2", "Fixed fluorescent 1", "Fixed fluorescent 2", "Hold current"]}, {["Auto", "Flicker-free 50 Hz", "Flicker-free 60 Hz", "Hold current"]}, {["None", "Prioritize frame rate", "Prioritize image quality"]}, {["Monochrome", "Color"]}] -> [_ _ _ _ _ w314]
          frame Default {
            w272 = FALSE ("Visible")
            w271 = FALSE ("Visible")
            n141 = property on="Motor" class="Clust (strict)"("Visible"=w271) -> ()  [unwired: 2 in, 2 out]
            n142 = property on="Test Ring" class="Ring (strict)"("Visible"=w271) -> ()  [unwired: 2 in, 2 out]
            n143 = property on="Rev/Fwd" class="Clust (strict)"("Visible"=w272) -> ()  [unwired: 2 in, 2 out]
            n144 = property on="On/Off" class="Bool (strict)"("Visible"=w272) -> ()  [unwired: 2 in, 2 out]
            n145 = property on="Test Slider" class="Slide (strict)"("Visible"=w272) -> ()  [unwired: 2 in, 2 out]
          }
          frame "Analog Out", "Motor", "PWM" {
            w278 = FALSE ("Visible")
            n146 = case shown="\"Analog Out\"" w277 {
              tunnel: [1.0 ("Value") -1.0 ("Value") 0.0 ("Value")] -> w276
              tunnel: [255.0 ("Value") 1.0 ("Value") 5.0 ("Value")] -> w275
              tunnel: [128.0 ("Value") 0.0 ("Value") 0.0 ("Value")] -> w274
              tunnel: [64.0 ("Value") 0.5 ("Value") 1.0 ("Value")] -> w273
              frame "PWM" {
              }
              frame "Motor", Default {
              }
              frame "Analog Out" {
              }
            }
            n147 = property on="Motor" class="Clust (strict)"("Visible"=TRUE) -> ()  [unwired: 2 in, 2 out]
            n148 = property on="Value" class="Slide (strict)"("Value"=w274, "Scale.Minimum"=w276, "Scale.Maximum"=w275, "Scale.Increment"=w273) -> ()  [unwired: 2 in, 2 out]
            n149 = property on="On/Off" class="Bool (strict)"("Visible"=w278) -> ()  [unwired: 2 in, 2 out]
            n150 = property on="Test Slider" class="Slide (strict)"("Visible"=w278) -> ()  [unwired: 2 in, 2 out]
            n151 = property on="Test Ring" class="Ring (strict)"("Visible"=w278) -> ()  [unwired: 2 in, 2 out]
            n152 = property on="Rev/Fwd" class="Clust (strict)"("Visible"=w278) -> ()  [unwired: 2 in, 2 out]
          }
          frame "Servo" {
            w294 = FALSE ("Visible")
            n153 = call <vilib>:"NT Read Number.vi"("Name"=w296) -> ("Numeric"=w295:dbl)  [unwired: 9 in, 1 out]
            n154 = property on="Test Slider" class="Slide (strict)"("Visible"=TRUE, "Scale.Maximum"=170.0 ("Scale.Range:Maximum")) -> ()  [unwired: 2 in, 2 out]
            n155 = local write "Test Slider"(w295) -> ()
            n156 = property on="Motor" class="Clust (strict)"("Visible"=w294) -> ()  [unwired: 2 in, 2 out]
            n157 = property on="Rev/Fwd" class="Clust (strict)"("Visible"=w294) -> ()  [unwired: 2 in, 2 out]
            n158 = property on="On/Off" class="Bool (strict)"("Visible"=w294) -> ()  [unwired: 2 in, 2 out]
            n159 = property on="Test Ring" class="Ring (strict)"("Visible"=w294) -> ()  [unwired: 2 in, 2 out]
          }
          frame "Relay", "Solenoid" {
            w297 = FALSE ("Visible")
            n160 = property on="Motor" class="Clust (strict)"("Visible"=w297) -> ()  [unwired: 2 in, 2 out]
            n161 = property on="Test Slider" class="Slide (strict)"("Visible"=w297) -> ()  [unwired: 2 in, 2 out]
            n162 = Search and Replace String(input string=w298, search string="/Value  **", replace string="/Direction") -> (result string=w304:string)  [unwired: 5 in, 3 out]
            n163 = property on="Test Ring" class="Ring (strict)"("Visible"=w297) -> ()  [unwired: 2 in, 2 out]
            n164 = call <vilib>:"NT Read String.vi"("Name"=w304) -> ("String"=w302:string)  [unwired: 9 in, 1 out]
            n165 = Equal?(x="Both directions", y=w302) -> (x = y?=w300:bool)
            n166 = Not(x=w300) -> (.not. x?=w301:bool)
            n167 = property on="Rev/Fwd" class="Clust (strict)"("Visible"=w300) -> ()  [unwired: 2 in, 2 out]
            n168 = property on="On/Off" class="Bool (strict)"("Visible"=w301, "Caption.Text"=w299) -> ()  [unwired: 2 in, 2 out]
          }
          frame "Compressor", "Digital Out" {
            w307 = FALSE ("Visible")
            # "Get direction and finish"
            n169 = property on="Motor" class="Clust (strict)"("Visible"=w307) -> ()  [unwired: 2 in, 2 out]
            n170 = property on="Test Slider" class="Slide (strict)"("Visible"=w307) -> ()  [unwired: 2 in, 2 out]
            n171 = property on="Test Ring" class="Ring (strict)"("Visible"=w307) -> ()  [unwired: 2 in, 2 out]
            n172 = property on="On/Off" class="Bool (strict)"("Visible"=TRUE, "Caption.Text"=w308) -> ()  [unwired: 2 in, 2 out]
            n173 = property on="Rev/Fwd" class="Clust (strict)"("Visible"=FALSE) -> ()  [unwired: 2 in, 2 out]
          }
          frame "Camera" {
            n174 = call <vilib>:"Get Last Path Segment.vi"("String in"=w315) -> ("String out"=w316:string)  [unwired: 10 in]
            n175 = property on="On/Off" class="Bool (strict)"("Visible"=FALSE) -> ()  [unwired: 2 in, 2 out]
            n176 = property on="Motor" class="Clust (strict)"("Visible"=FALSE) -> ()  [unwired: 2 in, 2 out]
            n177 = property on="Rev/Fwd" class="Clust (strict)"("Visible"=FALSE) -> ()  [unwired: 2 in, 2 out]
            n178 = case shown="\"White Balance  **\"" w316 {
              tunnel: w315 -> [w322 w331 w340 w349 w358 _ w364]
              tunnel: w314 -> [w320 w328 w337 w346 w355 _ _]
              frame "Size  **" {
                n179 = Index Array(array=w320) -> (element=w319:cluster{string[]})  [unwired: 1 in]
                n180 = call <vilib>:"NT Read String.vi"("Name"=w322) -> ("String"=w321:string)  [unwired: 9 in, 1 out]
                n181 = Unbundle(w319) -> (w317:string[])
                n182 = Match First String(2:w317, 3:w321) -> (0:w318:i32)  [unwired: 1 out]
                n183 = property on="Test Ring" class="Ring (strict)"("Value"=w318, "Strings []"=w317) -> ()  [unwired: 2 in, 2 out]
                n184 = property on="Test Ring" class="Ring (strict)"("Visible"=TRUE) -> ()  [unwired: 2 in, 2 out]
                n185 = property on="Test Slider" class="Slide (strict)"("Visible"=FALSE) -> ()  [unwired: 2 in, 2 out]
              }
              frame "White Balance  **" {
                n186 = Index Array(array=w328, index=1) -> (element=w329:cluster{string[]})
                n187 = call <vilib>:"NT Read String.vi"("Name"=w331) -> ("String"=w330:string)  [unwired: 9 in, 1 out]
                n188 = Unbundle(w329) -> (w326:string[])
                n189 = Match First String(2:w326, 3:w330) -> (0:w325:i32)  [unwired: 1 out]
                n190 = property on="Test Ring" class="Ring (strict)"("Value"=w325, "Strings []"=w326) -> ()  [unwired: 2 in, 2 out]
                n191 = property on="Test Ring" class="Ring (strict)"("Visible"=TRUE) -> ()  [unwired: 2 in, 2 out]
                n192 = property on="Test Slider" class="Slide (strict)"("Visible"=FALSE) -> ()  [unwired: 2 in, 2 out]
              }
              frame "Exposure  **" {
                n193 = Index Array(array=w337, index=2) -> (element=w338:cluster{string[]})
                n194 = call <vilib>:"NT Read String.vi"("Name"=w340) -> ("String"=w339:string)  [unwired: 9 in, 1 out]
                n195 = Unbundle(w338) -> (w334:string[])
                n196 = Match First String(2:w334, 3:w339) -> (0:w335:i32)  [unwired: 1 out]
                n197 = property on="Test Ring" class="Ring (strict)"("Value"=w335, "Strings []"=w334) -> ()  [unwired: 2 in, 2 out]
                n198 = property on="Test Ring" class="Ring (strict)"("Visible"=TRUE) -> ()  [unwired: 2 in, 2 out]
                n199 = property on="Test Slider" class="Slide (strict)"("Visible"=FALSE) -> ()  [unwired: 2 in, 2 out]
              }
              frame "Exposure Priority  **" {
                n200 = Index Array(array=w346, index=3) -> (element=w347:cluster{string[]})
                n201 = call <vilib>:"NT Read String.vi"("Name"=w349) -> ("String"=w348:string)  [unwired: 9 in, 1 out]
                n202 = Unbundle(w347) -> (w343:string[])
                n203 = Match First String(2:w343, 3:w348) -> (0:w344:i32)  [unwired: 1 out]
                n204 = property on="Test Ring" class="Ring (strict)"("Value"=w344, "Strings []"=w343) -> ()  [unwired: 2 in, 2 out]
                n205 = property on="Test Ring" class="Ring (strict)"("Visible"=TRUE) -> ()  [unwired: 2 in, 2 out]
                n206 = property on="Test Slider" class="Slide (strict)"("Visible"=FALSE) -> ()  [unwired: 2 in, 2 out]
              }
              frame "Color Enable  **" {
                n207 = Index Array(array=w355, index=4) -> (element=w356:cluster{string[]})
                n208 = call <vilib>:"NT Read String.vi"("Name"=w358) -> ("String"=w357:string)  [unwired: 9 in, 1 out]
                n209 = Unbundle(w356) -> (w352:string[])
                n210 = Match First String(2:w352, 3:w357) -> (0:w353:i32)  [unwired: 1 out]
                n211 = property on="Test Ring" class="Ring (strict)"("Value"=w353, "Strings []"=w352) -> ()  [unwired: 2 in, 2 out]
                n212 = property on="Test Ring" class="Ring (strict)"("Visible"=TRUE) -> ()  [unwired: 2 in, 2 out]
                n213 = property on="Test Slider" class="Slide (strict)"("Visible"=FALSE) -> ()  [unwired: 2 in, 2 out]
              }
              frame Default {
                n214 = property on="Test Ring" class="Ring (strict)"("Visible"=FALSE) -> ()  [unwired: 2 in, 2 out]
                n215 = property on="Test Slider" class="Slide (strict)"("Visible"=FALSE) -> ()  [unwired: 2 in, 2 out]
              }
              frame "Brightness  **", "Color Level  **", "Compression  **", "FPS  **", "Sharpness  **" {
                n216 = call <vilib>:"NT Read Number.vi"("Name"=w364) -> ("Numeric"=w363:dbl)  [unwired: 9 in, 1 out]
                n217 = local write "Test Slider"(w363) -> ()
                n218 = property on="Test Slider" class="Slide (strict)"("Visible"=TRUE, "Scale.Maximum"=100.0 ("Scale.Range:Maximum")) -> ()  [unwired: 2 in, 2 out]
                n219 = property on="Test Ring" class="Ring (strict)"("Visible"=FALSE) -> ()  [unwired: 2 in, 2 out]
              }
            }
          }
        }
        n220 = property on="Progress" class="Clust (strict)"("Visible"=FALSE) -> ()  [unwired: 2 in, 2 out]
      }
      event "Test Name": Mouse Enter {
        # "Populate the ring with the list of tests"
        n221 = event-data() -> ()  [unwired: 1 in, 1 out]
        n222 = call <vilib>:"NT Read String Array.vi"("Name"="TestMode/TestList") -> ("String Array"=w372:string[])  [unwired: 9 in, 1 out]
        n223 = Build Array (concatenate)("Select the test to run...", w372) -> (w371:string[])
        n224 = property on="Test Name" class="Ring (strict)"("Strings []"=w371) -> ()  [unwired: 2 in, 2 out]
      }
      event "Test Name": Value Change {
        w374 = FALSE ("Visible")
        # "Tell the robot the test name to run"
        n225 = event-data() -> ("NewVal"=w378:u16)  [unwired: 1 in]
        n226 = property on="Test Name" class="Ring (strict)"() -> ("Strings []"=w379:string[])  [unwired: 2 in, 2 out]
        n227 = local write "Progress"(T6 {"Test Progress"=0, "Test Progress Text"=""} ("Progress")) -> ()
        n228 = Index Array(array=w379, index=w378) -> (element=w377:string)
        n229 = call <vilib>:"NT Write String.vi"("String"=w377, "Name"="TestMode/TestName") -> ()  [unwired: 9 in, 1 out]
        n230 = property on="Progress" class="Clust (strict)"("Visible"=TRUE) -> ()  [unwired: 2 in, 2 out]
        n231 = property on="Motor" class="Clust (strict)"("Visible"=w374) -> ()  [unwired: 2 in, 2 out]
        n232 = property on="Test Slider" class="Slide (strict)"("Visible"=w374) -> ()  [unwired: 2 in, 2 out]
        n233 = property on="On/Off" class="Bool (strict)"("Visible"=w374) -> ()  [unwired: 2 in, 2 out]
        n234 = property on="Rev/Fwd" class="Clust (strict)"("Visible"=w374) -> ()  [unwired: 2 in, 2 out]
        n235 = property on="Test Ring" class="Ring (strict)"("Visible"=w374) -> ()  [unwired: 2 in, 2 out]
      }
      event "Select Auto": Mouse Enter {
        # "Populate the combo box with the list of autonomous options"
        n236 = event-data() -> ()  [unwired: 1 in, 1 out]
        n237 = call <vilib>:"NT Read String Array.vi"("Name"="Auto List") -> ("String Array"=w381:string[])  [unwired: 9 in, 1 out]
        n238 = property on="Select Auto" class="CmbBox"("Strings[]"=w381) -> ()  [unwired: 2 in, 2 out]
      }
      event "Select Auto": Value Change {
        # "User modified the Auto Selection. Write to NT variable so robot knows."
        n239 = event-data() -> ("NewVal"=w384:string)  [unwired: 1 in]
        n240 = call <vilib>:"NT Write String.vi"("String"=w384, "Name"="Auto Selector") -> ()  [unwired: 9 in, 1 out]
      }
      event "Command Selection": Value Change {
        # "Get the params and show in table"
        n241 = event-data() -> ("NewVal"=w390:i32)  [unwired: 1 in]
        n242 = property on="Command Selection" class="MCListbox (strict)"() -> ("ItemNames"=w388:string[][])  [unwired: 2 in, 2 out]
        n243 = call <vilib>:"WPI_DashboardUpdate Command Params.vi"("NewVal"=w390, "Commands"=w388, "Param Tbl"=w389) -> ()  [unwired: 8 in, 1 out]
      }
      event "Execute Command": Value Change {
        # "Started one, Unique ID holds\nresponse"
        n244 = event-data() -> ()  [unwired: 1 in, 1 out]
        n245 = property on="Command Selection" class="MCListbox (strict)"() -> ("ItemNames"=w401:string[][])  [unwired: 2 in, 2 out]
        n246 = Index Array(array=w401, index (row)="Command Selection", index (col)=0) -> (element=w399:string)
        n247 = call <vilib>:"Invoke Commands.vi"("Command Params"="Command Params", "Function Name"=w399) -> ("Params"=w395:u8, "Started"=w394:bool)  [unwired: 7 in, 1 out]
        n248 = Array Subset(array="Command Params", length (row)=w395) -> (w396:string[][])  [unwired: 3 in]
        n249 = Select(t="Executing" ("Cmd Status"), s=w394, f="" ("Cmd Status")) -> (s? t:f=→"Cmd Status":string)
      }
      event "Command Selection": Double Click {
        n250 = event-data() -> ("Row"=w409:i32)  [unwired: 1 in]
        n251 = property on="Command Selection" class="MCListbox (strict)"() -> ("ItemNames"=w412:string[][])  [unwired: 2 in, 2 out]
        n252 = local read "Command Params"() -> (w408:string[][])
        n253 = Index Array(array=w412, index (row)=w409, index (col)=0) -> (element=w410:string)
        n254 = call <vilib>:"Invoke Commands.vi"("Command Params"=w408, "Function Name"=w410) -> ("Params"=w407:u8, "Started"=w402:bool)  [unwired: 7 in, 1 out]
        n255 = Array Subset(array=w408, length (row)=w407) -> (w406:string[][])  [unwired: 3 in]
        n256 = Select(t="Executing" ("Cmd Status"), s=w402, f="" ("Cmd Status")) -> (s? t:f=w403:string)
        n257 = local write "Cmd Status"(w403) -> ()
      }
      event "CheckList": Double Click {
        # "Shift clears all"
        # "Update symbols on the listbox"
        n258 = event-data() -> ("PlatMods.Shift"=w414:bool, "Row"=w416:i32)  [unwired: 1 in]
        n259 = case shown="True" w414 {
          tunnel: w416 -> [w420 _]
          tunnel: 1 -> [w419 _]
          frame False {
            n260 = property on="CheckList" class="LstBox (strict)"() -> ("Item Symbols"=w418:i32[])  [unwired: 2 in, 2 out]
            n261 = Replace Array Subset(array=w418, new element=w419, index=w420) -> (w417:i32[])
            n262 = property on="CheckList" class="LstBox (strict)"("Item Symbols"=w417) -> ()  [unwired: 2 in, 2 out]
          }
          frame True {
            w421 = 0 ("Top Row")
            n263 = property on="CheckList" class="LstBox (strict)"() -> ("Number of Rows"=w423:u32)  [unwired: 2 in, 2 out]
            n264 = Initialize Array(0, w423) -> (w422:i32[])
            n265 = property on="CheckList" class="LstBox (strict)"("Top Row"=w421, "Value"=w421, "Item Symbols"=w422) -> ()  [unwired: 2 in, 2 out]
          }
        }
      }
      event "CheckList": Key Down {
        # "Update symbols on the listbox\nLeft and right keys check and uncheck"
        n266 = event-data() -> ("VKey"=w427:T21)  [unwired: 1 in]
        n267 = case shown="\"Left\", \"Right\"" w427 {
          selector: w427 -> [w432 _]
          tunnel: eventvkey."Left" ("VKey") -> [w430 _]
          frame "Left", "Right" {
            n268 = Equal?(x=w430, y=w432) -> (x = y?=w431:bool)
            n269 = Select(t=0, s=w431, f=1) -> (s? t:f=w433:i32)
            n270 = property on="CheckList" class="LstBox (strict)"() -> ("Item Symbols"=w436:i32[])  [unwired: 2 in, 2 out]
            n271 = Replace Array Subset(array=w436, new element=w433, index="CheckList") -> (w435:i32[])
            n272 = property on="CheckList" class="LstBox (strict)"("Item Symbols"=w435) -> ()  [unwired: 2 in, 2 out]
          }
          frame Default {
          }
        }
      }
      event "Motor.Enable": Value Change {
        # "When the test mode otor enable helper is set, update that\ntree row item's value"
        n273 = event-data() -> ("NewVal"=w442:bool)  [unwired: 1 in]
        n274 = Unbundle("Motor") -> ("Value"=w441:dbl)  [unwired: 1 out]
        n275 = Select(t=w441, s=w442, f=0.0) -> (s? t:f=w439:dbl)
        n276 = call <vilib>:"NT Write Number.vi"("Numeric"=w439, "Name"=w438) -> ()  [unwired: 9 in, 1 out]
      }
      event "Test Slider": Value Change {
        # "When the test mode slider helper is set, update that\ntree row item's value"
        n277 = event-data() -> ("NewVal"=w445:dbl)  [unwired: 1 in]
        n278 = call <vilib>:"NT Write Number.vi"("Numeric"=w445, "Name"=w446) -> ()  [unwired: 9 in, 1 out]
      }
      event "On/Off": Value Change {
        # "When the test mode on/off helper value is set, update that\ntree row item's value"
        n279 = event-data() -> ("NewVal"=w450:bool)  [unwired: 1 in]
        n280 = Boolean To (0,1)(Boolean=w450) -> (0, 1=w449:i16)
        n281 = call <vilib>:"NT Write Number.vi"("Numeric"=w449, "Name"=w448) -> ()  [unwired: 9 in, 1 out]
      }
      event "Rev/Fwd": Value Change {
        # "When the test mode helper value for relays is set, update that\ntree row item's value"
        n282 = event-data() -> ("NewVal.Forward"=w458:bool, "NewVal.Reverse"=w457:bool)  [unwired: 1 in]
        n283 = Boolean To (0,1)(Boolean=w458) -> (0, 1=w454:i16)
        n284 = Boolean To (0,1)(Boolean=w457) -> (0, 1=w456:i16)
        n285 = Negate(x=w456) -> (-x=w455:i16)
        n286 = Add(x=w454, y=w455) -> (x+y=w453:i16)
        n287 = call <vilib>:"NT Write Number.vi"("Numeric"=w453, "Name"=w452) -> ()  [unwired: 9 in, 1 out]
      }
      event "Test Ring": Value Change {
        # "When a test mode helper value is selected from the ring,\nset the tree item's variable to the string value"
        n288 = event-data() -> ("NewVal"=w462:u16)  [unwired: 1 in]
        n289 = property on="Test Ring" class="Ring (strict)"() -> ("Strings []"=w463:string[])  [unwired: 2 in, 2 out]
        n290 = Index Array(array=w463, index=w462) -> (element=w461:string)
        n291 = call <vilib>:"NT Write String.vi"("String"=w461, "Name"=w460) -> ()  [unwired: 9 in, 1 out]
      }
      event "Rec Mode": Value Change {
        # "Update globals for recording mode and path to read log from.\nClear when logging and let NetworkTables set path for vision to\nuse."
        n292 = event-data() -> ("NewVal"=w474:enum32{"Stop", "Record", "Playback"})  [unwired: 1 in]
        n293 = global write "WPI_DashboardLogging Global.vi" "Logging Filename"(path "") -> ()
        n294 = global write "WPI_DashboardLogging Global.vi" "Recording"(w474) -> ()
        n295 = case shown="\"Playback\"" w474 {
          tunnel: w473 -> [_ w476 w485]
          tunnel: [_ _ w484] -> w471
          tunnel: [_ _ w483] -> _
          tunnel: w469 -> [_ _ w481]
          tunnel: cluster{i32, i32} {-250, 170} -> [_ _ w480]
          tunnel: [_ _ T22 {"Image Size"=TRUE, "Image Type"=TRUE, "Pixel Value"=TRUE, "ROI Information"=TRUE, "Zoom Factor"=FALSE} ("Image Information Shown:All Elements")] -> w464
          tunnel: [_ _ TRUE ("Zoom Factor")] -> w465
          tunnel: w467 -> [_ _ w477]
          frame Default {
          }
          frame "Stop", "Record" {
            # "Place Window too"
            n296 = invoke class="VI" method="FP.Close"(reference=w476) -> (reference out=w475:refnum<vi>)  [unwired: 2 in, 2 out]
            n297 = invoke class="VI" method="Abort VI"(reference=w475) -> ()  [unwired: 2 in, 3 out]
          }
          frame "Playback" {
            n298 = call "Open Playback Panel.vi"("Offset"=w480, "DB VI Ref"=w481, "Playback in"=w485) -> ("Playback out"=w482:refnum<vi>)  [unwired: 8 in]
            n299 = register-events(w482, w477) -> (reference out=w484:refnum<event-registration>, error out=w483:errorcluster)  [unwired: 2 in]
          }
        }
        n300 = property on="Camera Image Right" class="ImageControl"("Image Information Shown"=w464, "Image Information Visible"=w465) -> ()  [unwired: 2 in, 2 out]
        n301 = property on="Camera Image" class="ImageControl"("Image Information Shown"=w464, "Image Information Visible"=w465) -> ()  [unwired: 2 in, 2 out]
        n302 = call <vilib>:"WPI_DashboardNT Log FieldName Cache.vi"("Operation"=enum16{"Lookup/Add", "Index", "Clear"}."Clear") -> ()  [unwired: 8 in, 3 out]
      }
      event Panel Close {
        w487 = enum32{"Stop", "Record", "Playback"}."Stop" ("Rec Mode")
        # "Playback window has been closed, abort"
        n303 = event-data() -> ()  [unwired: 1 in, 4 out]
        n304 = local write "Rec Mode"(w487) -> ()
        n305 = global write "WPI_DashboardLogging Global.vi" "Recording"(w487) -> ()
      }
      event Panel Close {
        # "Abort playback window and ourself"
        n306 = event-data() -> ()  [unwired: 1 in, 4 out]
        n307 = invoke class="VI" method="FP.Close"(reference=w491) -> (reference out=w490:refnum<vi>)  [unwired: 2 in, 2 out]
        n308 = invoke class="VI" method="Abort VI"(reference=w490) -> (error out=w489:errorcluster)  [unwired: 2 in, 2 out]
        n309 = invoke class="VI" method="Abort VI"(error in=w489) -> ()  [unwired: 2 in, 3 out]
      }
      event User Event {
        n310 = event-data() -> ("IDs"=w498:cluster{"RPC field ID":u16, "Unique ID":u16}, "String"=w497:string)  [unwired: 1 in]
        n311 = Bundle("IDs"=w498, "String"=w497) -> (w496:T9)  [unwired: 1 in]
        n312 = call <vilib>:"Retrieve RPC Response.vi"("RPC Response"=w496) -> ("Output"=w494:string[][])  [unwired: 10 in]
        n313 = Build Array (concatenate)(w492, w494) -> (w493:string[][])
        n314 = local write "Command Params"(w493) -> ()
        n315 = local write "Cmd Status"("" ("Cmd Status")) -> ()
      }
      event "Tree": Double Click {
        n316 = event-data() -> ("PlatMods"=w504:T25, "Tag"=w501:string)  [unwired: 1 in]
        n317 = Unbundle(w504) -> ("Shift"=w503:bool)  [unwired: 4 out]
        n318 = String Subset(string=w501, length (rest)=1 ("length (rest)")) -> (substring=w500:string)  [unwired: 1 in]
        n319 = Not(x=w503) -> (.not. x?=w502:bool)
        n320 = case shown="\"/\"" w500 {
          tunnel: w501 -> [_ w507]
          tunnel: w502 -> [_ w506]
          frame Default {
          }
          frame "/" {
            n321 = call <vilib>:"NT Update Persistence.vi"("Persistence"=w506, "Name"=w507) -> ()  [unwired: 9 in, 1 out]
          }
        }
      }
    }
  }
  n322 = while {
    tunnel: w66 -> [w509]
    i -> [w512]
    stop <- FALSE stop-if-true
    n323 = Wait (ms)(milliseconds to wait=u32 100) -> ()  [unwired: 1 out]
    n324 = case shown="\"Playback\"" "Rec Mode" {
      tunnel: w512 -> [_ _ w527]
      tunnel: [u32 2829099 ("Base Color") u32 11141120 ("Target Color") w516] -> w508
      frame "Stop", Default {
        # "Reset the color, extra updates don't cost much"
      }
      frame "Record" {
      }
      frame "Playback" {
        # "Playback"
        n325 = Quotient & Remainder(x=w527, y=u32 50 ("milliseconds to wait")) -> (x-y*floor(x/y)=w523:u32)  [unwired: 1 out]
        n326 = Divide(x=w523, y=u32 50 ("milliseconds to wait")) -> (x/y=w520:dbl)
        n327 = Multiply(x=6.283185307179586, y=w520) -> (x*y=w525:dbl)
        n328 = Sine(x=w525) -> (sin(x)=w524:dbl)
        n329 = Absolute Value(x=w524) -> (abs(x)=w517:dbl)
        n330 = call "Interpolate RGB Color.vi"("Proportion"=w517, "Target Color"=u32 30976, "Base Color"=u32 2829099) -> ("Result Color"=w516:u32)  [unwired: 8 in]
      }
    }
    n331 = property class="Pane"(reference=w509, "PaneColor"=w508) -> ()  [unwired: 1 in, 2 out]
  }
  n332 = local write "Dashboard Tab"(T2."Drive" ("Dashboard Tab")) -> ()
  n333 = property on="On/Off" class="Bool (strict)"("Visible"=w37) -> ()  [unwired: 2 in, 2 out]
  n334 = property on="Motor" class="Clust (strict)"("Visible"=w37) -> ()  [unwired: 2 in, 2 out]
  n335 = property on="Progress" class="Clust (strict)"("Visible"=w37) -> ()  [unwired: 2 in, 2 out]
  n336 = property on="Test Ring" class="Ring (strict)"("Visible"=w37) -> ()  [unwired: 2 in, 2 out]
  n337 = property on="Rev/Fwd" class="Clust (strict)"("Visible"=w37) -> ()  [unwired: 2 in, 2 out]
  n338 = while {
    tunnel: u16 1741 ("timeout ms (25000)") -> [w529]
    stop <- FALSE stop-if-true
    n339 = TCP Create Listener(10:w529) -> (0:w528:errorcluster, 3:w530:refnum<k5>)  [unwired: 4 in, 1 out]
    n340 = case shown="No Error" w528 {
      selector: w528 -> [w532 _]
      tunnel: w530 -> [w533 _]
      frame No Error {
        n341 = while {
          tunnel: w533 -> [w536]
          tunnel: w532 -> [w535]
          stop <- FALSE stop-if-true
          n342 = TCP Wait On Listener(8:w535, 11:w536) -> (0:w537:errorcluster, 4:w538:refnum<k5>)  [unwired: 2 in, 3 out]
          n343 = local write "TCP"(w538) -> ()
          n344 = case shown="No Error" w537 {
            frame No Error {
            }
            frame Error {
              n345 = Wait (ms)(milliseconds to wait=u32 1000) -> ()  [unwired: 1 out]
            }
          }
        }
      }
      frame Error {
        n346 = Wait (ms)(milliseconds to wait=u32 1000) -> ()  [unwired: 1 out]
      }
    }
  }
  n347 = local write "Command Selection"(u16 0 ("milliseconds to wait")) -> ()
  n348 = local write "Command Params"(string[][] [] ("Command Params")) -> ()
  n349 = global write "WPI_DashboardLogging Global.vi" "Recording"(w60) -> ()
  n350 = local write "Rec Mode"(w60) -> ()
  n351 = call <vilib>:"NT Write String.vi"("String"="Select Auto", "Name"="Auto Selector") -> ()  [unwired: 9 in, 1 out]
  n352 = control-ref of="Tree"() -> (w1:refnum<vi>)
  n353 = call "Variable Graphing.vi"("Tree Refnum"=w1) -> ()  [unwired: 10 in]
  n354 = disable-structure shown="Disabled" {
    frame Disabled {
      n355 = call <vilib>:"WPI_DriverStationGame Specific Data.vi"() -> ()  [unwired: 11 in, 1 out]
    }
    frame Enabled {
    }
  }
  n356 = call "FRC Color Processing.vi"() -> ()  [unwired: 12 in]
